vi "BD Testing.vi"() -> ()   [LabVIEW 2018]
panel:
  out "Ref Data":cluster{"Num":i32}
  out "Array":string[](array[string])
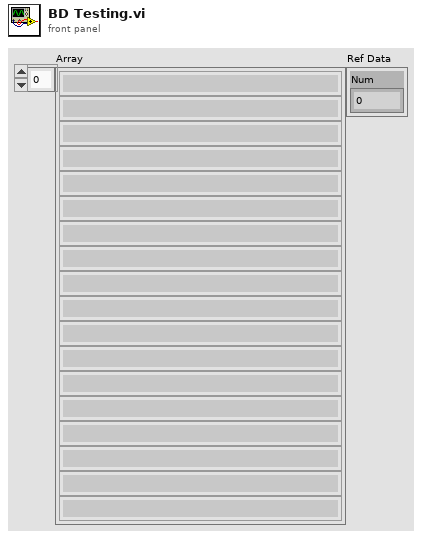
[diagram p1: front panel]
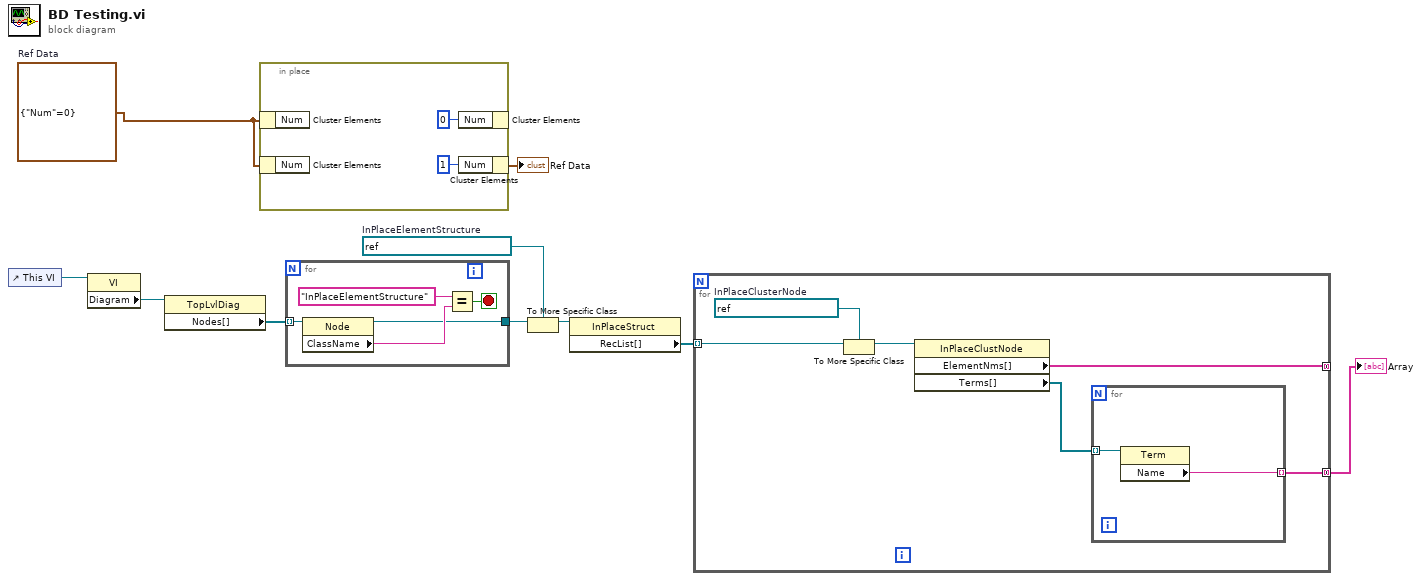
[diagram p0: block diagram]
diagram:
  w6 = refnum<vi> refnum  # InPlaceElementStructure
  w2 = cluster{"Num":i32} {"Num"=0}  # Ref Data
  n1 = control-ref of="This VI"() -> (w10:refnum<vi>)
  n2 = property on="Property Node" class="VI"(reference=w10) -> ("Diagram"=w9:refnum<vi>)  [unwired: 1 in, 2 out]
  n3 = property on="Property Node" class="TopLvlDiag"(reference=w9) -> ("Nodes[]"=w8:refnum<vi>[])  [unwired: 1 in, 2 out]
  n4 = in-place {
    n5 = in-place-cluster #1(w2) -> ()  [unwired: 1 out]
    n6 = in-place-cluster #2(w2) -> ()  [unwired: 1 out]
    n7 = in-place-cluster #1("Num"=0) -> ()  [unwired: 1 out]
    n8 = in-place-cluster #2("Num"=1) -> (→"Ref Data":cluster{"Num":i32})
  }
  n9 = for {
    tunnel: w8 -> [w17] mode=indexing
    tunnel: [w13] -> w7
    stop <- w14 stop-if-true
    n10 = property class="Node"(reference=w17) -> (reference out=w13:refnum<vi>, "ClassName"=w15:string)  [unwired: 1 in, 1 out]
    n11 = Equal?(x="InPlaceElementStructure", y=w15) -> (x = y?=w14:bool)
  }
  n12 = To More Specific Class(target class=w6, reference=w7) -> (specific class reference=w5:refnum<vi>)  [unwired: 1 in, 1 out]
  n13 = property class="InPlaceStruct"(reference=w5) -> ("RecList[]"=w4:refnum<vi>[])  [unwired: 1 in, 2 out]
  n14 = for {
    tunnel: w4 -> [w23] mode=indexing
    tunnel: [w22] -> _ mode=concatenating
    tunnel: [w18] -> w3 mode=concatenating
    w19 = refnum<vi> refnum  # InPlaceClusterNode
    n15 = To More Specific Class(target class=w19, reference=w23) -> (specific class reference=w20:refnum<vi>)  [unwired: 1 in, 1 out]
    n16 = property class="InPlaceClustNode"(reference=w20) -> ("ElementNms[]"=w22:string[], "Terms[]"=w21:refnum<vi>[])  [unwired: 1 in, 2 out]
    n17 = for {
      tunnel: w21 -> [w25] mode=indexing
      tunnel: [w24] -> w18 mode=indexing
      n18 = property class="Term"(reference=w25) -> ("Name"=w24:string)  [unwired: 1 in, 2 out]
    }
  }
  "Array" <- w3
